vi "LIA_Host.vi"() -> ()   [LabVIEW 2012]
uses:
  <vilib>/userdefined/High Color/nirio_resource_hc.ctl
  <vilib>/LabVIEW Targets/FPGA/cRIO/shared/nicrio_ModuleControls/nicrio_cRIO-9233_DataRatesRing.ctl
  <vilib>/FPGAPlugInAG/PCI-7831R/niLvFpga_Open_PCI-7831R.vi
  <vilib>/FPGAPlugInAG/PCI-7831R/niLvFpga_Download_PCI-7831R.vi
  <vilib>/FPGAPlugInAG/PCI-7831R/niLvFpga_Reset_PCI-7831R.vi
  <vilib>/Utility/error.llb/Error Cluster From Error Code.vi
  <vilib>/FPGAPlugInAG/PCI-7831R/niLvFpga_Run_PCI-7831R.vi
  <vilib>/RVI Host/nirviSupport.llb/nirviErrorClusterFromErrorCode.vi
  <vilib>/rvi/errors/niLvFpgaAdjustHostInterfaceError.vi
  <vilib>/FPGAPlugInAG/PCI-7831R/niLvFpga_Close_PCI-7831R.vi
  <vilib>/rvi/interface/nirviOpenFPGA/nirviOpenFPGA.xnode
  FPGA Bitfiles/LIA_FPGATarget_LIAFPGA_UBXKlbf10UU.lvbitx
  LIA_FPGA.vi
  <vilib>/rvi/interface/nirviMethod/nirviMethod.xnode
  <vilib>/rvi/interface/nirviReadWriteControl/nirviReadWriteControl.xnode
  <vilib>/rvi/interface/nirviCloseFPGA/nirviCloseFPGA.xnode
  NiFpgaLv.dll
  <vilib>/rvi/errors/niLvFpgaMergeErrorWithErrorCode.vi
  <vilib>/FPGAPlugInAG/PCI-7831R/niLvFpga_ConfigureFifo_PCI-7831R.vi
  <vilib>/rvi/interface/nirviMethod/StockFPGA_InlinedMethodWaitForSingleIRQ.vi
  <vilib>/FPGAPlugInAG/PCI-7831R/niLvFpga_WaitOnIrq_PCI-7831R.vi
  <vilib>/FPGAPlugInAG/PCI-7831R/niLvFpga_AcknowledgeIrq_PCI-7831R.vi
  <vilib>/FPGAPlugInAG/PCI-7831R/niLvFpga_ReadFifo_PCI-7831R.vi
panel:
  out "Locked?":bool
  out "Locked Frequency [Hz]":dbl
  out "Phase [degree]":dbl
  out "Amplitude [V]":dbl
  in  "Data Rate":T1=2 items=["50.000 kS/s (NI 9233)"=2, "33.333 kS/s (NI 9233)"=3, "25.000 kS/s (NI 9233)"=34, "16.667 kS/s (NI 9233)"=35, "12.500 kS/s (NI 9233)"=36, "10.000 kS/s (NI 9233)"=37, "  8.333 kS/s (NI 9233)"=38, "  7.143 kS/s (NI 9233)"=39, "  6.250 kS/s (NI 9233)"=40, "  5.556 kS/s (NI 9233)"=41, "  5.000 kS/s (NI 9233)"=42, "  4.545 kS/s (NI 9233)"=43, "  4.167 kS/s (NI 9233)"=44, "  3.846 kS/s (NI 9233)"=45, "  3.571 kS/s (NI 9233)"=46, "  3.333 kS/s (NI 9233)"=47, "  3.125 kS/s (NI 9233)"=48, "  2.941 kS/s (NI 9233)"=49, "  2.778 kS/s (NI 9233)"=50, "  2.632 kS/s (NI 9233)"=51, "  2.500 kS/s (NI 9233)"=52, "  2.381 kS/s (NI 9233)"=53, "  2.273 kS/s (NI 9233)"=54, "  2.174 kS/s (NI 9233)"=55, "  2.083 kS/s (NI 9233)"=56, "  2.000 kS/s (NI 9233)"=57]
  out "Waveform Graph":sgl[][](graph)
  in  "stop":bool
  out "channel Q":dbl
  out "channel I":dbl
  in  "Nominal Freqency [Hz]":dbl=1000.0 format="%#.8g"
  in  "Filter Rolloff":enum16{"20 dB", "40 dB", "60 dB", "80 dB"}(ring)
  in  "Time Constant [s]":dbl=1.0 min=0.0 format="%.2f"
  in  "Resource Name":T2
  out "calib":cluster{"LSB Weight":u32, "Offset":i32}
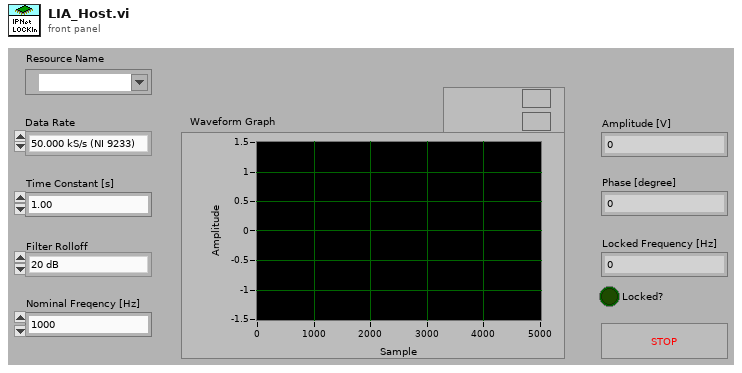
[diagram p1: front panel]
types:
  T1 = typedef "nicrio_cRIO-9233_DataRatesRing.ctl" = u8
  T2 = typedef "nirio_resource_hc.ctl" = tag
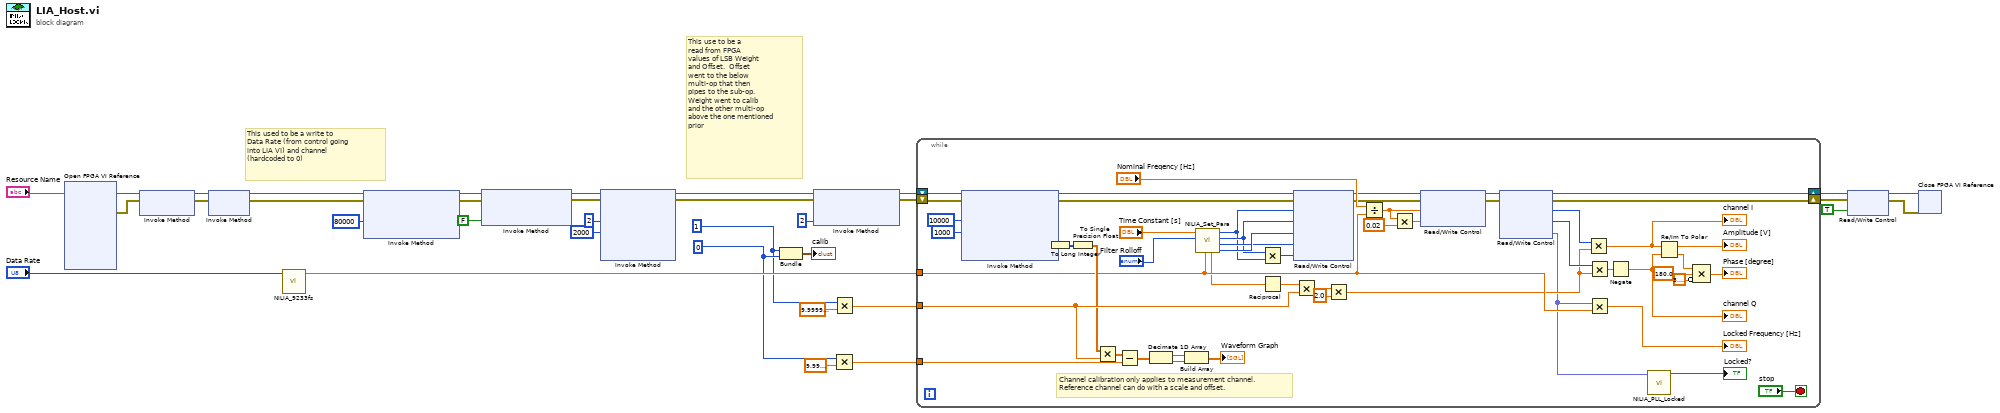
[diagram p0: block diagram]
diagram:
  w2 = 1
  w3 = 0
  # "This use to be a\nread from FPGA\nvalues of LSB Weight\nand Offset.  Offset\nwent to the below\nmulti-op that then\npipes to the sub-op.\nWeight went to calib\nand the other multi-op\nabove the one mentioned\nprior"
  # "This used to be a write to\nData Rate (from control going\ninto LIA VI) and channel \n(hardcoded to 0)"
  n1 = xnode "Open FPGA VI Reference"("resource name"="Resource Name") -> ("FPGA VI Reference Out"=w34:refnum<k20>, "error out"=w33:errorcluster)  [unwired: 1 in]
  n2 = xnode "Invoke Method"("FPGA VI Reference In"=w34, "error in"=w33) -> ("FPGA VI Reference Out"=w32:refnum<k20>, "error out"=w31:errorcluster)
  n3 = xnode "Invoke Method"("FPGA VI Reference In"=w32, "error in"=w31) -> ("FPGA VI Reference Out"=w6:refnum<k20>, "error out"=w1:errorcluster)
  n4 = call "NILIA_9233fs.vi"("Data Rate"="Data Rate") -> ("fs"=w8:dbl)  [unwired: 10 in]
  n5 = xnode "Invoke Method"("FPGA VI Reference In"=w6, "error in"=w1, "Requested Depth"=u32 80000 ("Depth")) -> ("FPGA VI Reference Out"=w22:refnum<k20>, "error out"=w21:errorcluster)  [unwired: 1 out]
  n6 = xnode "Invoke Method"("FPGA VI Reference In"=w22, "error in"=w21, "Wait Until Done (F)"=FALSE) -> ("FPGA VI Reference Out"=w27:refnum<k20>, "error out"=w26:errorcluster)
  n7 = xnode "Invoke Method"("FPGA VI Reference In"=w27, "error in"=w26, "IRQ Number(s)"=2, "Timeout (ms)"=2000) -> ("FPGA VI Reference Out"=w5:refnum<k20>, "error out"=w4:errorcluster)  [unwired: 2 out]
  n8 = Bundle(w2, w3) -> (→"calib":cluster{i32, i32})  [unwired: 1 in]
  n9 = xnode "Invoke Method"("FPGA VI Reference In"=w5, "error in"=w4, "IRQ Number(s)"=2) -> ("FPGA VI Reference Out"=w20:refnum<k20>, "error out"=w19:errorcluster)
  n10 = Multiply(x=w3, y=sgl 1e-09) -> (x*y=w9:sgl)
  n11 = Multiply(x=w2, y=sgl 1e-12) -> (x*y=w17:sgl)
  n12 = while {
    shift-right: [w84] -> w16
    shift-left: w20 -> [w76]
    shift-right: [w83] -> w15
    shift-left: w19 -> [w75]
    tunnel: w17 -> [w71]
    tunnel: w9 -> [w72]
    tunnel: w8 -> [w65]
    stop <- "stop" stop-if-true
    # "Channel calibration only applies to measurement channel.\nReference channel can do with a scale and offset."
    n13 = xnode "Invoke Method"("FPGA VI Reference In"=w76, "error in"=w75, "Number of Elements"=u32 10000, "Timeout (ms)"=1000) -> ("FPGA VI Reference Out"=w74:refnum<k20>, "error out"=w73:errorcluster, "Data"=w78:i32[])  [unwired: 1 out]
    n14 = To Long Integer(number=w78) -> (32bit integer=w77:i32[])
    n15 = To Single Precision Float(number=w77) -> (single precision float=w70:sgl[])
    n16 = Multiply(x=w70, y=w71) -> (x*y=w79:sgl[])
    n17 = Subtract(x=w79, y=w72) -> (x-y=w67:sgl[])
    n18 = Decimate 1D Array(w67) -> (w68:sgl[], w69:sgl[])
    n19 = Build Array(w68, w69) -> (→"Waveform Graph":sgl[][])
    n20 = call "NILIA_Set_Para.vi"("fs"=w65, "rolloff"="Filter Rolloff", "TC [sec]"="Time Constant [s]") -> ("3rd stages"=w51:i32, "3rd decimation"=w50:i32, "2nd decimation"=w49:i32, "1st decimation"=w48:i32, "corr"=w45:dbl)  [unwired: 4 in]
    n21 = Multiply(x=w49, y=w48) -> (x*y=w52:i32)
    n22 = Reciprocal(x=w45) -> (1/x=w44:dbl)
    n23 = xnode "Read/Write Control"("FPGA VI Reference In"=w74, "error in"=w73, "dec1"=w48, "dec2"=w49, "stages"=w51, "decimation"=w50, "dec"=w52) -> ("FPGA VI Reference Out"=w55:refnum<k20>, "error out"=w56:errorcluster)
    n24 = Multiply(x=w44, y=w71) -> (x*y=w43:dbl)
    n25 = Multiply(x=w43, y=2.0) -> (x*y=w39:dbl)
    n26 = Divide(x="Nominal Freqency [Hz]", y=w65) -> (x/y=w37:dbl)
    n27 = Multiply(x=w37, y=0.02) -> (x*y=w53:dbl)
    n28 = xnode "Read/Write Control"("FPGA VI Reference In"=w55, "error in"=w56, "nominal freq"=w37, "K"=w53) -> ("FPGA VI Reference Out"=w47:refnum<k20>, "error out"=w46:errorcluster)
    n29 = xnode "Read/Write Control"("FPGA VI Reference In"=w47, "error in"=w46) -> ("FPGA VI Reference Out"=w84:refnum<k20>, "error out"=w83:errorcluster, "channelI"=w41:i64, "channelQ"=w40:i64, "f"=w36:fxp<+/-,32,0>)
    n30 = Multiply(x=w41, y=w39) -> (x*y=w64:dbl)
    "channel I" <- w64
    n31 = Multiply(x=w40, y=w39) -> (x*y=w38:dbl)
    n32 = Multiply(x=w36, y=w65) -> (x*y=→"Locked Frequency [Hz]":dbl)
    n33 = Negate(x=w38) -> (-x=w63:dbl)
    "channel Q" <- w63
    n34 = call "NILIA_PLL_Locked.vi"("f"=w36) -> ("locked"=→"Locked?":bool)  [unwired: 10 in]
    n35 = Re/Im To Polar(2:w63, 3:w64) -> (0:w61:dbl, 1:→"Amplitude [V]":dbl)
    n36 = Compound Arithmetic op=MULTIPLY(w61, 180.0 ("value"), invert 3.141592653589793) -> (→"Phase [degree]":dbl)
  }
  n37 = xnode "Read/Write Control"("FPGA VI Reference In"=w16, "error in"=w15, "stop"=TRUE) -> ("FPGA VI Reference Out"=w13:refnum<k20>, "error out"=w12:errorcluster)
  n38 = xnode "Close FPGA VI Reference"("FPGA VI Reference In"=w13, "error in"=w12) -> ()  [unwired: 1 out]
